vi "0816147.vi"() -> ()   [LabVIEW 2021]
panel:
  out "num":T1
  in  "OK Button":bool
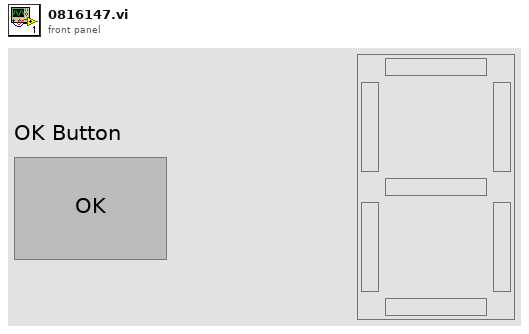
[diagram p1: front panel]
types:
  T1 = cluster{"Boolean 1":bool, "Boolean 2":bool, "Boolean 3":bool, "Boolean 4":bool, "Boolean 5":bool, "Boolean 6":bool, "Boolean 7":bool}
  T2 = cluster{"[0]":bool, "[1]":bool, "[2]":bool, "[3]":bool, "[4]":bool, "[5]":bool, "[6]":bool}
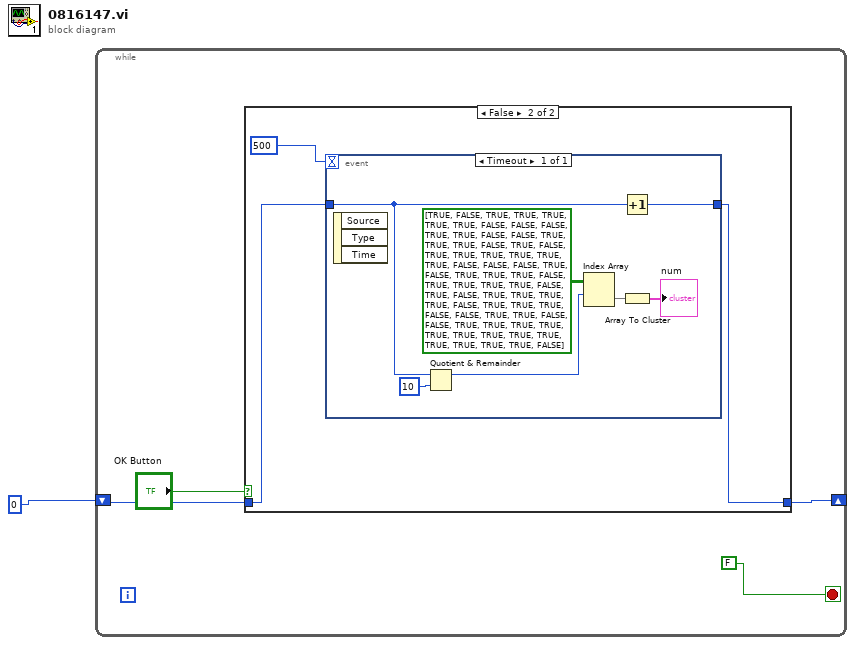
[diagram p0: block diagram]
diagram:
  n1 = while {
    shift-right: [w3] -> _
    shift-left: 0 -> [w4]
    stop <- FALSE stop-if-true
    n2 = case shown="False" "OK Button" {
      tunnel: w4 -> [w6 w9]
      tunnel: [w6 w8] -> w3
      frame True {
      }
      frame False {
        n3 = event shown="[0] Timeout" {
          selector: _ -> [_]
          dyn-events: _ -> [_]
          timeout: 500 -> [_]
          tunnel: w9 -> [w12]
          tunnel: [w10] -> w8
          event Timeout {
            n4 = event-data() -> ()  [unwired: 1 in, 3 out]
            n5 = Quotient & Remainder(x=w12, y=10) -> (x-y*floor(x/y)=w16:i32)  [unwired: 1 out]
            n6 = Index Array(array=bool[][] [[TRUE, FALSE, TRUE, TRUE, TRUE, TRUE, TRUE], [FALSE, FALSE, FALSE, TRUE, TRUE, FALSE, FALSE], [TRUE, TRUE, TRUE, FALSE, TRUE, FALSE, TRUE], [TRUE, TRUE, TRUE, TRUE, TRUE, FALSE, FALSE], [FALSE, TRUE, FALSE, TRUE, TRUE, TRUE, FALSE], [TRUE, TRUE, TRUE, TRUE, FALSE, TRUE, FALSE], [TRUE, TRUE, TRUE, TRUE, FALSE, TRUE, TRUE], [TRUE, FALSE, FALSE, TRUE, TRUE, FALSE, FALSE], [TRUE, TRUE, TRUE, TRUE, TRUE, TRUE, TRUE], [TRUE, TRUE, TRUE, TRUE, TRUE, TRUE, FALSE]], index (row)=w16) -> (element=w15:bool[])  [unwired: 1 in]
            n7 = Increment(x=w12) -> (x+1=w10:i32)
            n8 = Array To Cluster(array=w15) -> (cluster=→"num":T2)
          }
        }
      }
    }
  }
